vi "set_env_variable.vi"(6 "Value":string, 7 "Environment Variable Name":string="labview_llm_openai_key") -> (0 "error out":errorcluster)   [LabVIEW 2020, in "env_variables.lvlib"]
uses:
  env_variables.lvlib
  <vilib>/Utility/config.llb/Write Key (String).vi
  <vilib>/Utility/config.llb/NI_LVConfig.lvlib
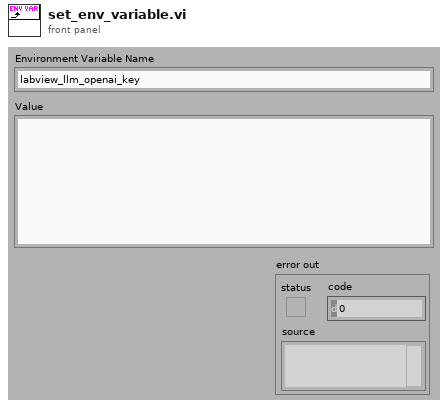
[diagram p1: front panel]
types:
  T1 = typedef "NI_LVConfig.lvlib/Config Data RefNum.ctl" = refnum<k1>
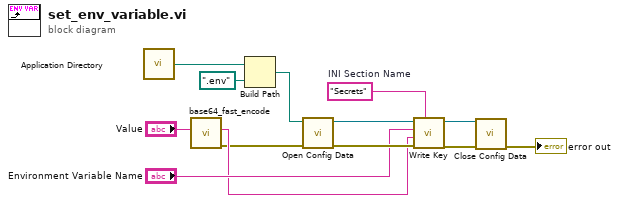
[diagram p0: block diagram]
diagram:
  w12 = "Secrets"  # INI Section Name
  n1 = call <vilib>:"Application Directory.vi"() -> ("Application Directory"=w10:path)
  n2 = call "base64_fast_encode.vi"("string in (not encoded)"="Value") -> ("error out"=w1:errorcluster, "string out (base64-encoded)"=w2:string)  [unwired: 9 in]
  n3 = Build Path(base path=w10, name or relative path=path ".env") -> (appended path=w8:path)
  n4 = call <vilib>:"Open Config Data.vi"("error in (no error)"=w1, "configuration file path"=w8) -> ("error out"=w13:errorcluster, "refnum"=w11:T1)  [unwired: 7 in, 1 out]
  n5 = call-poly <vilib>:"Write Key.vi"("section"=w12, "error in (no error)"=w13, "value"=w2, "key"="Environment Variable Name", "refnum"=w11) -> ("error out"=w5:errorcluster, "refnum out"=w6:T1)  [unwired: 4 in, 1 out]
  n6 = call <vilib>:"Close Config Data.vi"("error in (no error)"=w5, "refnum"=w6) -> ("error out"=→"error out":errorcluster)  [unwired: 8 in, 1 out]
